vi "Handle GET.vi"(8 "error in (no error)":errorcluster, 10 "parameter":string, 11 "Instrument in":refnum<class "Instrument.lvclass">) -> (0 "error out":errorcluster, 2 "data out":variant, 3 "Instrument out":refnum<class "Instrument.lvclass">)   [LabVIEW 2019, in "Instrument.lvclass"]
uses:
  Instrument.lvclass
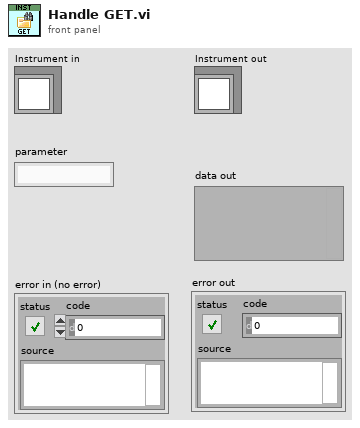
[diagram p1: front panel]
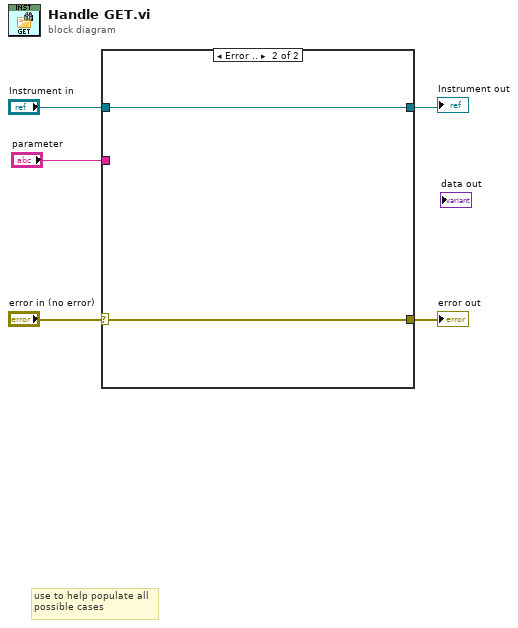
[diagram p0: block diagram]
diagram:
  # "use to help populate all\npossible cases"
  n1 = case shown="Error .." "error in (no error)" {
    selector: "error in (no error)" -> [w6 w8]
    tunnel: [w7 w9] -> w5
    tunnel: "Instrument in" -> [w7 w9]
    tunnel: [w6 w8] -> w3
    tunnel: "parameter" -> [_ _]
    frame No Error {
      # "child must override"
    }
    frame Error {
    }
  }
  "Instrument out" <- w5
  "error out" <- w3
